vi "PVCAM_GetLastError_Safe.vi"() -> (3 "return type":i16)   [LabVIEW 2021]
uses:
  pvcam64.dll
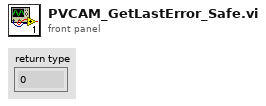
[diagram p1: front panel]
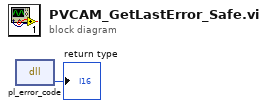
[diagram p0: block diagram]
diagram:
  n1 = dll-call lib="pvcam64.dll" fn="pl_error_code"() -> ("return type"=→"return type":i16)  [unwired: 3 in, 2 out]
